vi "Cmd to R_W - Synchronous.vi"(8 "error in":errorcluster, 10 "write buffer":string, 11 "Serial IO in":refnum<class "Serial IO.lvclass">) -> (0 "error out":errorcluster, 2 "read buffer":string, 3 "Serial IO out":refnum<class "Serial IO.lvclass">)   [LabVIEW 2015, in "Serial IO.lvclass"]
doc: "In most instances, retrieval of data from a serial port is commenced with a write. This VI writes to the port and then waits for a response. Depending on the configuration, the VISA read will be based on:\n1) A specified amount of time for bytes to become available before perfomring a read on that port. These parameters (as well as the port enumeration) are located in the superclass.\n2) For the end as defined by the parameter ASRL End In.\nIf (2) is not defined in the device configuration then the execution of this VI will proceed using the wait for bytes loop found in case 0.\n\n<B>This VI is reentrant to allow access to the different ports that different devices might be communicating with simultaneously.</B>"
uses:
  Serial IO.lvclass
  Serial IO.lvclass/Serial IO.ctl
  <vilib>/Platform/TimedLoop/XDataNode/timing_clust.ctl
  <vilib>/Platform/TimedLoop/XDataNode/nitl_modes.ctl
  <vilib>/Platform/TimedLoop/XDataNode/wakeup.ctl
  <vilib>/Platform/TimedLoop/XDataNode/XDataNode.xnode
  <vilib>/Platform/TimedLoop/XDataNode/XDNodeRunTimeDep.lvlib
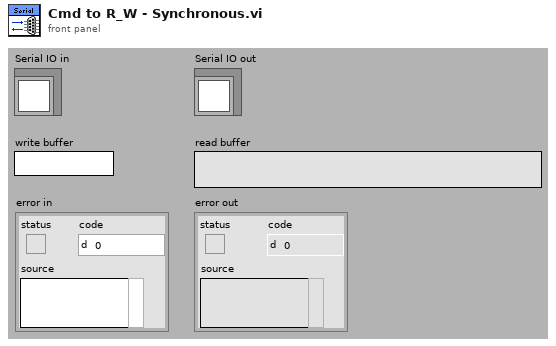
[diagram p1: front panel]
types:
  T1 = typedef "XDNodeRunTimeDep.lvlib/timing_clust.ctl" = cluster{"Expected End [f-1]":u64, "Actual End [f-1]":u64, "Finished Late? [f-1]":bool, "Expected End [i-1]":u64, "Actual End [i-1]":u64, "Finished Late? [i-1]":bool, "Expected Start [i]":u64, "Actual Start [i]":u64, "Expected Start [f]":u64, "Actual Start [f]":u64, "Source Name":string, "Structure Name":string, "Period":i64, "Deadline":i64, "Offset":i64, "Start":i64, "Priority":i32, "Timeout":i32, "Mode":T2, "Wakeup Reason":T3, "Error":errorcluster, "Source Type":string, "Secondary Source Type":string, "Global End Time":u64, "Global Start Time":u64, "Frame Duration":u64, "Iteration Duration":u64, "Assigned CPU":i32, "I/O Scan Engine Mode":u32}
  T2 = typedef "XDNodeRunTimeDep.lvlib/nitl_modes.ctl" = enum32{"No Change", "Process missed periods, maintain original phase", "Discard missed periods, maintain original phase", "Process missed periods, ignore original phase", "Discard missed periods, ignore original phase"}
  T3 = typedef "XDNodeRunTimeDep.lvlib/wakeup.ctl" = enum32{"Normal", "Aborted", "Asynchronous wakeup", "Timing source error", "Timed loop error", "Timeout"}
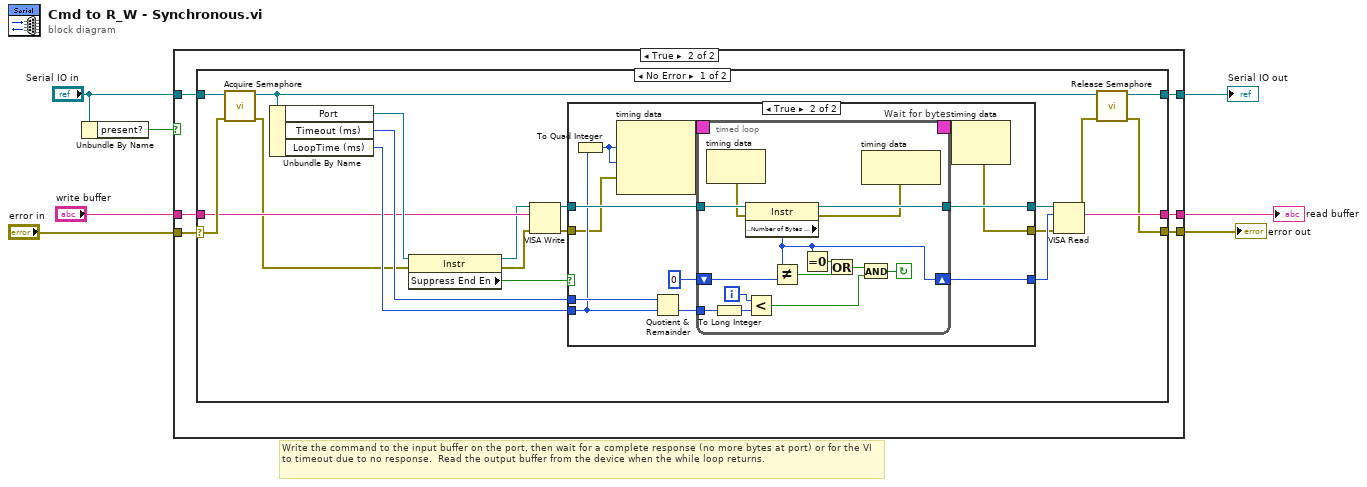
[diagram p0: block diagram]
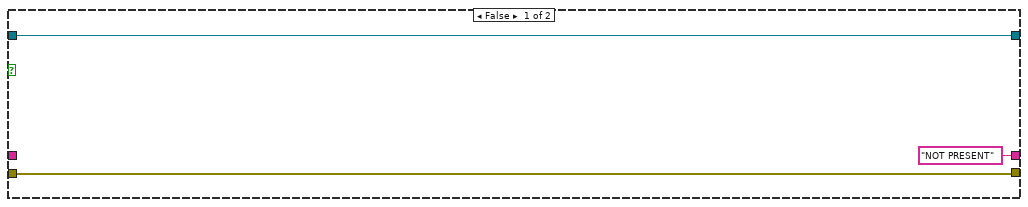
[diagram p2: hidden frame]
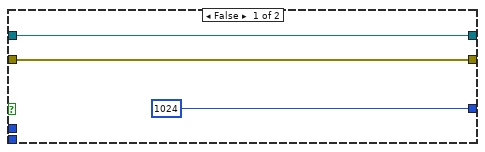
[diagram p3: hidden frame]
diagram:
  # "Write the command to the input buffer on the port, then wait for a complete response (no more bytes at port) or for the VI to timeout due to no response.  Read the output buffer from the device when the while loop returns."
  n1 = Unbundle By Name("Serial IO in") -> ("present?"=w1:bool)
  n2 = case shown="True" w1 {
    tunnel: [w10 w16] -> w7
    tunnel: "error in" -> [w8 w15]
    tunnel: [w8 w14] -> w5
    tunnel: ["NOT PRESENT" ("read buffer") w13] -> w4
    tunnel: "write buffer" -> [_ w12]
    tunnel: "Serial IO in" -> [w10 w11]
    frame False {
    }
    frame True {
      n3 = case shown="No Error" w15 {
        selector: w15 -> [w25 w79]
        tunnel: [w21 w79] -> w14
        tunnel: [w23 w78] -> w16
        tunnel: [w29 _] -> w13
        tunnel: w11 -> [w26 w78]
        tunnel: w12 -> [w20 _]
        frame No Error {
          n4 = call "Acquire Semaphore.vi"("error in"=w25, "Serial IO in"=w26) -> ("error out"=w19:errorcluster, "Serial IO out"=w24:refnum<class "Serial IO.lvclass">)  [unwired: 8 in]
          n5 = Unbundle By Name(w24) -> ("Port"=w28:refnum<visa-resource-name>, "Timeout (ms)"=w33:u32, "LoopTime (ms)"=w32:u32)
          n6 = property class="Instr"(reference=w28, error in=w19) -> (reference out=w18:refnum<visa-resource-name>, error out=w17:errorcluster, "Suppress End En"=w27:bool)
          n7 = VISA Write(VISA resource name=w18, write buffer=w20, error in (no error)=w17) -> (VISA resource name out=w36:refnum<visa-resource-name>, error out=w31:errorcluster)  [unwired: 1 out]
          n8 = case shown="True" w27 {
            tunnel: w36 -> [w38 w49]
            tunnel: [w38 w48] -> w35
            tunnel: [u32 1024 w47] -> w34
            tunnel: w33 -> [_ w46]
            tunnel: w32 -> [_ w45]
            tunnel: w31 -> [w39 w44]
            tunnel: [w39 w43] -> w30
            frame False {
            }
            frame True {
              n9 = To Quad Integer(1:w45) -> (0:w40:i64)
              n10 = node-c288(w40, w40, w44) -> (w51:T1)
              n11 = Quotient & Remainder(x=w46, y=w45) -> (floor(x/y)=w42:u32)  [unwired: 1 out]
              n12 = timed-loop "Wait for bytes" {
                tunnel: w49 -> [w65]
                tunnel: [w64] -> w48
                tunnel: w42 -> [w53]
                shift-right: [w56] -> w47
                shift-left: u32 0 -> [w57]
                timing: w51 -> [_]
                timing-out: [_] -> w50
                i -> [w63]
                stop <- w62 continue-if-true
                n13 = node-c288() -> (w55:errorcluster)  [unwired: 1 in]
                n14 = To Long Integer(number=w53) -> (32bit integer=w52:i32)
                n15 = property class="Instr"(reference=w65, error in=w55) -> (reference out=w64:refnum<visa-resource-name>, error out=w54:errorcluster, "Serial Settings:Number of Bytes at Serial Port"=w56:u32)
                n16 = Less?(x=w63, y=w52) -> (x < y?=w61:bool)
                n17 = Not Equal?(x=w56, y=w57) -> (x != y?=w60:bool)
                n18 = Equal To 0?(x=w56) -> (x = 0?=w59:bool)
                n19 = Or(x=w59, y=w60) -> (x .or. y?=w58:bool)
                n20 = And(x=w58, y=w61) -> (x .and. y?=w62:bool)
                n21 = node-c288(w54) -> ()  [unwired: 1 out]
              }
              n22 = node-c288(w50) -> (w43:errorcluster)
            }
          }
          n23 = VISA Read(VISA resource name=w35, byte count=w34, error in (no error)=w30) -> (read buffer=w29:string, error out=w22:errorcluster)  [unwired: 2 out]
          n24 = call "Release Semaphore.vi"("error in (no error)"=w22, "Serial IO in"=w24) -> ("error out"=w21:errorcluster, "Serial IO out"=w23:refnum<class "Serial IO.lvclass">)  [unwired: 8 in]
        }
        frame Error {
        }
      }
    }
  }
  "Serial IO out" <- w7
  "error out" <- w5
  "read buffer" <- w4
